vi "Set position FM (SubVI).vi"(0 "VISA Refnum in":refnum<visa-resource-name>, 2 "Позиция, мкм":i32, 3 "error in":errorcluster, 4 "pos_z":dbl) -> (6 "set_pos_z":dbl, 7 "error out":errorcluster)   [LabVIEW 2018]
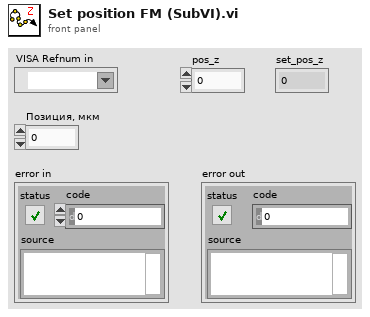
[diagram p1: front panel]
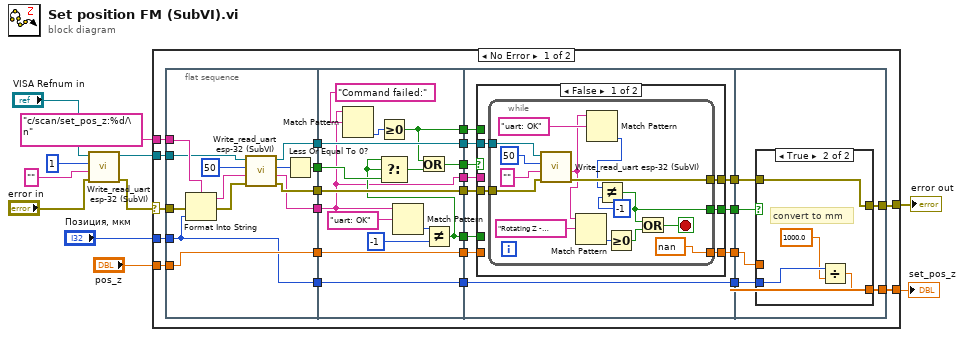
[diagram p0: block diagram]
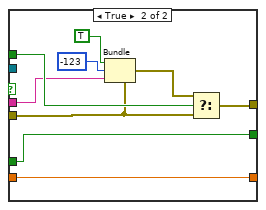
[diagram p2: hidden frame]
diagram:
  n1 = call "Write_read_uart esp-32 (SubVI).vi"("error in (no error)"="error in", "write buffer"="", "milliseconds to wait"=u32 1, "VISA Refnum in"="VISA Refnum in") -> ("error out 4"=w2:errorcluster, "VISA resource name out"=w1:refnum<visa-resource-name>)  [unwired: 2 out]
  n2 = case shown="No Error" w2 {
    selector: w2 -> [w34 w118]
    tunnel: [w33 w118] -> w11
    tunnel: "c/scan/set_pos_z:%d/\n" ("format string") -> [w36 _]
    tunnel: "Позиция, мкм" -> [w35 _]
    tunnel: "pos_z" -> [w30 w117]
    tunnel: [w29 w117] -> w7
    tunnel: w1 -> [w12 _]
    frame No Error {
      n3 = flat-sequence {
        tunnel: w36 -> [w41]
        tunnel: w35 -> [w38]
        tunnel: w34 -> [w45]
        tunnel: [w48] -> w26
        tunnel: [w44] -> w24
        tunnel: [w42] -> w22
        tunnel: w30 -> [w40]
        tunnel: [w38] -> w21
        tunnel: [w40] -> w19
        tunnel: [w39] -> w17
        tunnel: w12 -> [w37]
        tunnel: w26 -> [w64]
        tunnel: [w64] -> w25
        tunnel: w24 -> [w63]
        tunnel: [w63] -> w23
        tunnel: w22 -> [w57]
        tunnel: w21 -> [w62]
        tunnel: [w62] -> w20
        tunnel: w19 -> [w61]
        tunnel: [w61] -> w18
        tunnel: w17 -> [w50]
        tunnel: [w56] -> w16
        tunnel: [w53] -> w15
        tunnel: [w51] -> w14
        tunnel: [w50] -> w13
        tunnel: w25 -> [w74]
        tunnel: w23 -> [w75]
        tunnel: [w72] -> w32
        tunnel: [w71] -> w31
        tunnel: w20 -> [w70]
        tunnel: [w70] -> w28
        tunnel: w18 -> [w69]
        tunnel: [w68] -> w27
        tunnel: w16 -> [w67]
        tunnel: w15 -> [w73]
        tunnel: w14 -> [w66]
        tunnel: w13 -> [w65]
        tunnel: [w110] -> w33
        tunnel: w32 -> [w109]
        tunnel: w31 -> [w108]
        tunnel: [w107] -> w29
        tunnel: w28 -> [w106]
        tunnel: w27 -> [w105]
        frame #0 {
          n4 = Format Into String(format string=w41, error in=w45, w38) -> (resulting string=w47:string, error out=w46:errorcluster)  [unwired: 1 in]
          n5 = call "Write_read_uart esp-32 (SubVI).vi"("error in (no error)"=w46, "write buffer"=w47, "milliseconds to wait"=u32 50, "VISA Refnum in"=w37) -> ("error out 4"=w48:errorcluster, "read buffer"=w39:string, "read bite"=w43:u32, "VISA resource name out"=w44:refnum<visa-resource-name>)
          n6 = Less Or Equal To 0?(x=w43) -> (x <= 0?=w42:bool)
        }
        frame #1 {
          n7 = Match Pattern(string=w50, regular expression="Command failed:") -> (offset past match=w52:i32)  [unwired: 1 in, 3 out]
          n8 = Greater Or Equal To 0?(x=w52) -> (x >= 0?=w51:bool)
          n9 = Match Pattern(string=w50, regular expression="uart: OK") -> (offset past match=w58:i32)  [unwired: 1 in, 3 out]
          n10 = Not Equal?(x=w58, y=-1 ("offset past match")) -> (x != y?=w56:bool)
          n11 = Select(t=w56, s=w56, f=w57) -> (s? t:f=w54:bool)
          n12 = Or(x=w51, y=w54) -> (x .or. y?=w53:bool)
        }
        frame #2 {
          n13 = case shown="False" w73 {
            tunnel: w74 -> [w80 w97]
            tunnel: w75 -> [w79 _]
            tunnel: [w78 w101] -> w71
            tunnel: [w77 w103] -> w72
            tunnel: [w76 w104] -> w68
            tunnel: w69 -> [_ w104]
            tunnel: w67 -> [_ w103]
            tunnel: w66 -> [_ w102]
            tunnel: w65 -> [_ w98]
            frame False {
              n14 = while {
                tunnel: w80 -> [w93]
                tunnel: w79 -> [w92]
                tunnel: [w88] -> w78
                tunnel: [w86] -> w77
                tunnel: [nan] -> w76
                stop <- w89 stop-if-true
                n15 = call "Write_read_uart esp-32 (SubVI).vi"("error in (no error)"=w93, "write buffer"="", "milliseconds to wait"=u32 50, "VISA Refnum in"=w92) -> ("error out 4"=w88:errorcluster, "read buffer"=w83:string)  [unwired: 2 out]
                n16 = Match Pattern(string=w83, regular expression="Rotating Z - stopped!") -> (offset past match=w84:i32)  [unwired: 1 in, 3 out]
                n17 = Match Pattern(string=w83, regular expression="uart: OK") -> (offset past match=w87:i32)  [unwired: 1 in, 3 out]
                n18 = Not Equal?(x=w87, y=-1 ("offset past match")) -> (x != y?=w86:bool)
                n19 = Greater Or Equal To 0?(x=w84) -> (x >= 0?=w82:bool)
                n20 = Or(x=w86, y=w82) -> (x .or. y?=w89:bool)
              }
            }
            frame True {
              n21 = Bundle(cluster=w97, "status"=TRUE, "code"=-123, "source"=w98) -> (w96:errorcluster)
              n22 = Select(t=w96, s=w102, f=w97) -> (s? t:f=w101:errorcluster)
            }
          }
        }
        frame #3 {
          n23 = case shown="True" w109 {
            tunnel: w108 -> [w112 w116]
            tunnel: [w112 w116] -> w110
            tunnel: [w111 w114] -> w107
            tunnel: w106 -> [_ w115]
            tunnel: w105 -> [w111 _]
            frame False {
            }
            frame True {
              # "convert to mm"
              n24 = Divide(x=w115, y=1000.0 ("x")) -> (x/y=w114:dbl)
            }
          }
        }
      }
    }
    frame Error {
    }
  }
  "set_pos_z" <- w7
  "error out" <- w11
